vi "1 - Conversor de Temperatura.vi"(1 "Entrada":dbl, 2 "(F) C -> F\n(T) F -> C":bool) -> (0 "Saída":dbl)   [LabVIEW 2020]
panel:
  # "C -> F"
  # "F -> C"
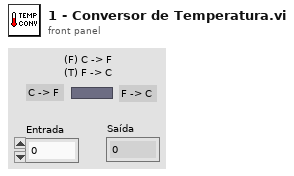
[diagram p1: front panel]
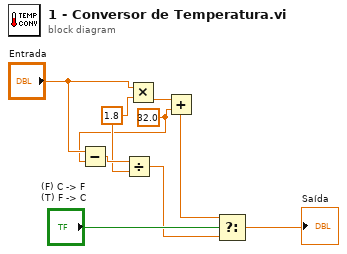
[diagram p0: block diagram]
diagram:
  w1 = 32.0
  w2 = 1.8
  n1 = Subtract(x="Entrada", y=w1) -> (x-y=w4:dbl)
  n2 = Divide(x=w4, y=w2) -> (x/y=w3:dbl)
  n3 = Multiply(x="Entrada", y=w2) -> (x*y=w7:dbl)
  n4 = Add(x=w7, y=w1) -> (x+y=w6:dbl)
  n5 = Select(t=w6, s="(F) C -> F\n(T) F -> C", f=w3) -> (s? t:f=→"Saída":dbl)
